vi "Add Child Items to Tree.vi"(8 "error in (no error)":errorcluster, 10 "Express VI Type in":refnum<class "Express VI Type.lvclass">, 11 "Tree Ref in":refnum<vi>) -> (0 "error out":errorcluster, 2 "Express VI Type out":refnum<class "Express VI Type.lvclass">, 3 "Tree Ref out":refnum<vi>)   [LabVIEW 2020, in "Peek Window.lvlib" / "Express VI Type.lvclass"]
uses:
  Express VI Type.lvclass
  Symbols Enum.ctl
  Express VI Type.lvclass/Express VI Type.ctl
  Standard VI Type/Standard VI Type.lvclass/Standard VI Type.ctl
  Standard VI Type/Read Full Qualified Name.vi
  Implementation VI Type/Implementation VI Type.lvclass
  D:/Code/VI-Peek/source/Peek Window/VI Types/Standard VI Type/Standard VI Type.lvclass
  Peek Window.lvlib
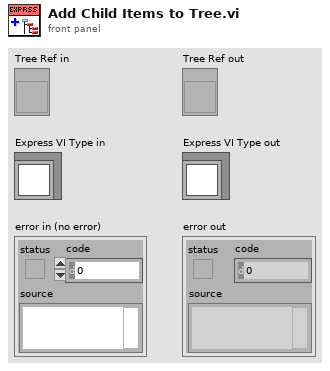
[diagram p1: front panel]
types:
  T1 = typedef "Peek Window.lvlib/Symbols Enum.ctl" = enum16{"<Blank>", "Implementation Mark", "Standard VI", "Dynamic Dispatch VI", "Malleable VI", "Polymorphic VI", "Missing VI", "Express VI"}
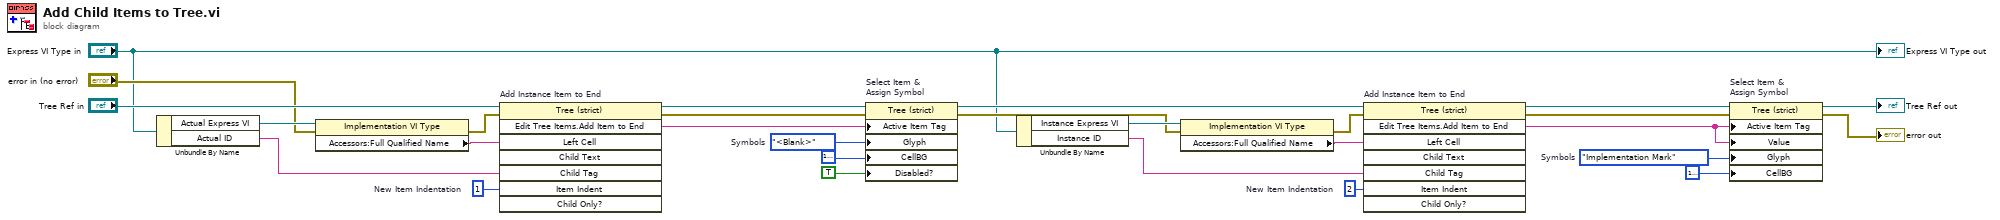
[diagram p0: block diagram]
diagram:
  w9 = Symbols_Enum."Implementation Mark"  # Symbols
  w10 = 2  # New Item Indentation
  w26 = Symbols_Enum."<Blank>"  # Symbols
  w25 = 1  # New Item Indentation
  n1 = Unbundle By Name("Express VI Type in") -> ("Actual Express VI"=w22:refnum<class "Implementation VI Type.lvclass">, "Actual ID"=w17:string)
  n2 = property class="Implementation VI Type"(reference=w22, error in="error in (no error)") -> (error out=w19:errorcluster, "Accessors:Full Qualified Name"=w20:string)  [unwired: 1 out]
  n3 = invoke on="Add Instance Item to End" class="Tree (strict)" method="Edit Tree Items.Add Item to End"(reference="Tree Ref in", error in=w19, "Left Cell"=w20, "Child Tag"=w17, "Item Indent"=w25) -> (reference out=w27:refnum<vi>, error out=w28:errorcluster, "Edit Tree Items:Add Item to End"=w21:string)  [unwired: 3 in, 5 out]
  n4 = property on="Select Item &\nAssign Symbol" class="Tree (strict)"(reference=w27, error in=w28, "Active Item Tag"=w21, "Glyph"=w26, "CellBG"=u32 16777238, "Disabled?"=TRUE) -> (reference out=w5:refnum<vi>, error out=w7:errorcluster)
  n5 = Unbundle By Name("Express VI Type in") -> ("Instance Express VI"=w12:refnum<class "Implementation VI Type.lvclass">, "Instance ID"=w16:string)
  n6 = property class="Implementation VI Type"(reference=w12, error in=w7) -> (error out=w15:errorcluster, "Accessors:Full Qualified Name"=w14:string)  [unwired: 1 out]
  n7 = invoke on="Add Instance Item to End" class="Tree (strict)" method="Edit Tree Items.Add Item to End"(reference=w5, error in=w15, "Left Cell"=w14, "Child Tag"=w16, "Item Indent"=w10) -> (reference out=w4:refnum<vi>, error out=w8:errorcluster, "Edit Tree Items:Add Item to End"=w13:string)  [unwired: 3 in, 5 out]
  n8 = property on="Select Item &\nAssign Symbol" class="Tree (strict)"(reference=w4, error in=w8, "Active Item Tag"=w13, "Value"=w13, "Glyph"=w9, "CellBG"=u32 16777238) -> (reference out=→"Tree Ref out":refnum<vi>, error out=→"error out":errorcluster)
  "Express VI Type out" <- "Express VI Type in"
